vi "initialize save.vi"(0 "Period [s]":i64, 7 "cRio data path":path=path "C:/data/LicorData") -> (8 "VI-data Save":T1={"Dateipfad save data"=path "", "file ref"=refnum, "number"=0, "Period [s]"=240, "Fehler (Ausgang)"={"status"=FALSE, "code"=0, "source"=""}})   [LabVIEW 2010, in "Licor-Steuerung.lvlib"]
uses:
  Licor-Steuerung.lvlib
  VI-data Save.ctl
  util/util.lvlib
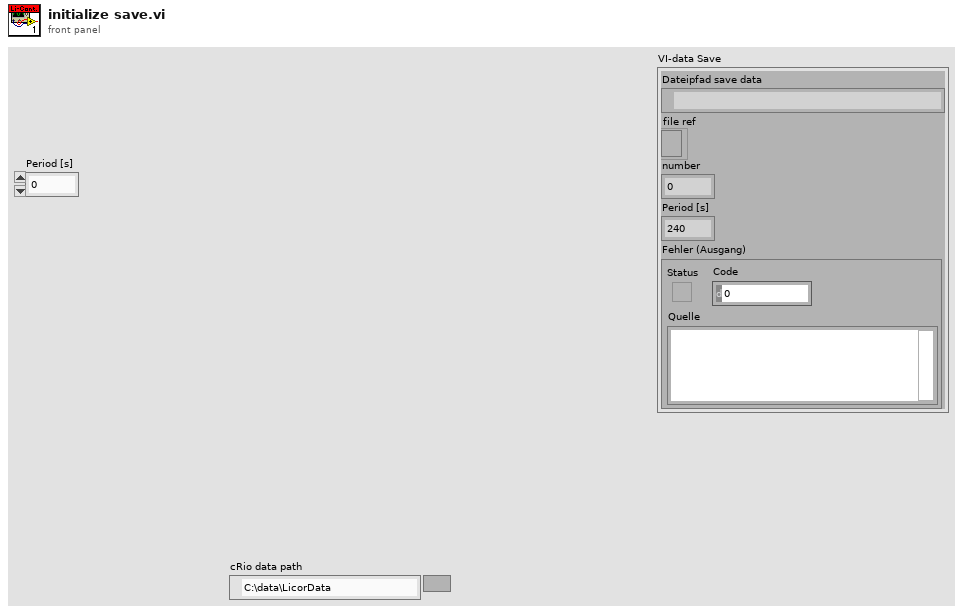
[diagram p1: front panel]
types:
  T1 = typedef "Licor-Steuerung.lvlib/VI-data Save.ctl" = cluster{"Dateipfad save data":path, "file ref":refnum<file>, "number":i64, "Period [s]":i64, "Fehler (Ausgang)":errorcluster}
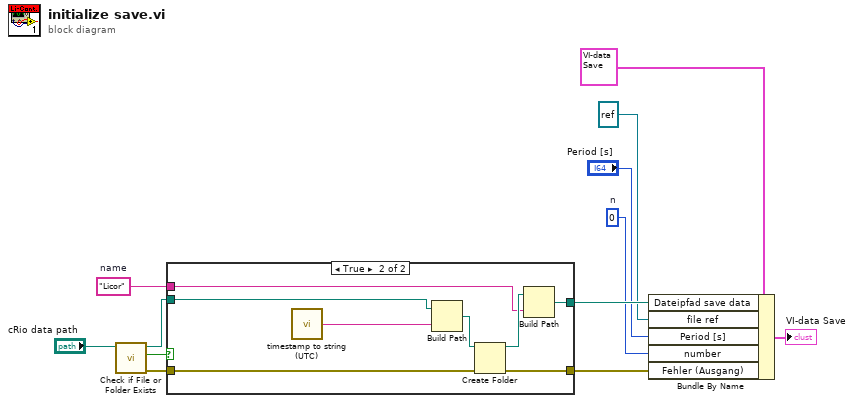
[diagram p0: block diagram]
diagram:
  w3 = i64 0  # n
  w9 = "Licor"  # name
  n1 = call <vilib>:"Check if File or Folder Exists.vi"("path"="cRio data path") -> ("error out"=w11:errorcluster, "file or folder exists?"=w12:bool, "dup path"=w10:path)  [unwired: 8 in]
  n2 = case shown="True" w12 {
    tunnel: [w14 w19] -> w4
    tunnel: w11 -> [w14 w20]
    tunnel: [w13 w16] -> w6
    tunnel: w10 -> [w13 w22]
    tunnel: w9 -> [_ w17]
    frame False {
    }
    frame True {
      n3 = call "timestamp to string (UTC).vi"() -> ("date/time string (UTC)"=w15:string)  [unwired: 14 in, 1 out]
      n4 = Build Path(base path=w22, name or relative path=w15) -> (appended path=w21:path)
      n5 = Create Folder(path (use dialog)=w21, error in=w20) -> (created path=w18:path, error out=w19:errorcluster)  [unwired: 1 in, 1 out]
      n6 = Build Path(base path=w18, name or relative path=w17) -> (appended path=w16:path)
    }
  }
  n7 = Bundle By Name(cluster=T1 {"Dateipfad save data"=path "", "file ref"=refnum, "number"=0, "Period [s]"=240, "Fehler (Ausgang)"={"status"=FALSE, "code"=0, "source"=""}} ("Eingangs-Cluster"), "Dateipfad save data"=w6, "file ref"=refnum<file> refnum ("y"), "Period [s]"="Period [s]", "number"=w3, "Fehler (Ausgang)"=w4) -> (→"VI-data Save":T1)
